vi "AdminLogInSearchHistory(SubVI).vi"() -> ()   [LabVIEW 2013]
uses:
  <vilib>/addons/database/Connection.llb/DB Tools Open Connec (String).vi
  <vilib>/addons/database/_DB Variant To Data/Database Variant To Data.xnode
  <vilib>/addons/database/NI_Database_API.lvlib
panel:
  in  "Search another student":bool
  in  "Confirm":bool
  in  "Student Admin No:":string
  in  "Go Back":bool
  out "Student Admin No: 2":string
  out "Array 2":string[][](array[string])
  out "AdminNo.Accepted?":string
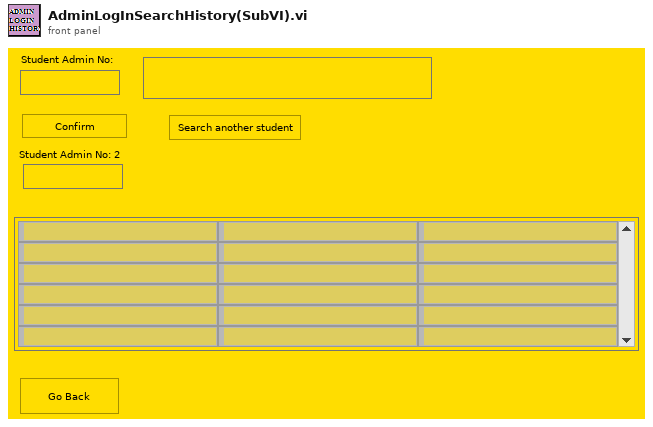
[diagram p1: front panel]
types:
  T1 = enum8{"Enabled", "Disabled", "Disabled and Grayed Out"}
  T2 = typedef "NI_Database_API.lvlib/Conn ObjectReference.ctl" = refnum<k1>
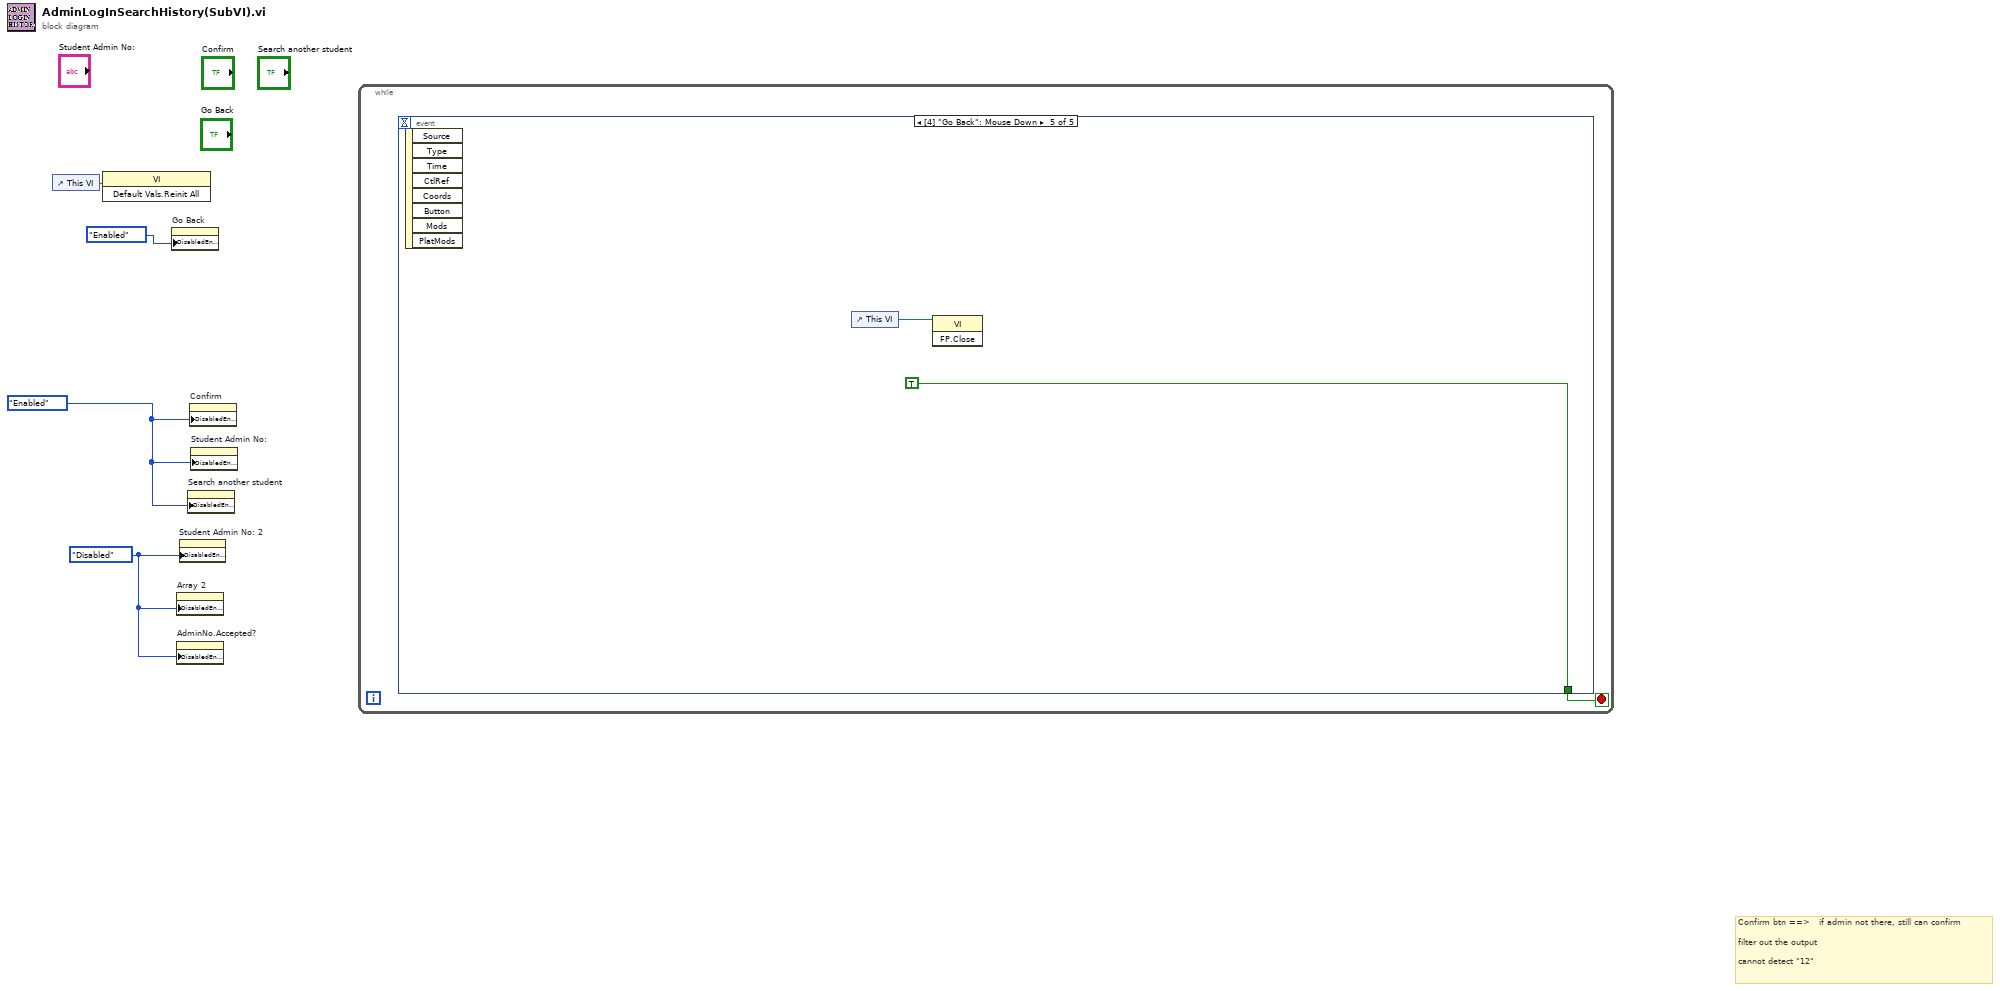
[diagram p0: block diagram]
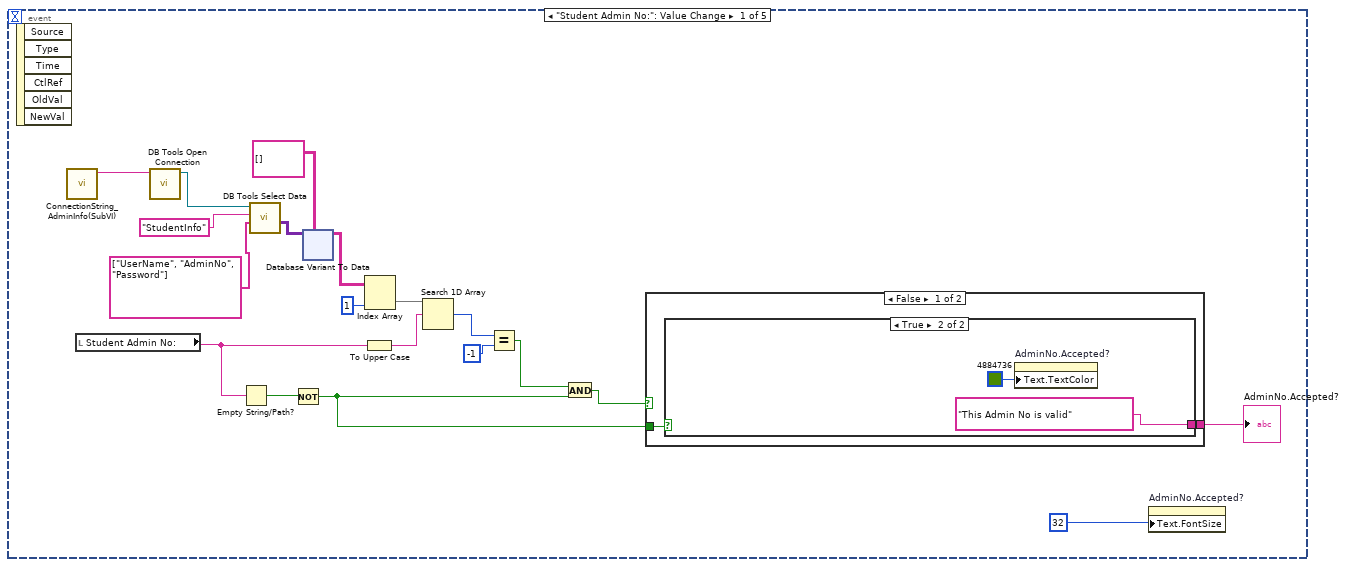
[diagram p2: hidden frame]
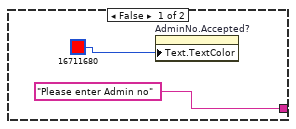
[diagram p3: hidden frame]
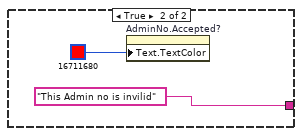
[diagram p4: hidden frame]
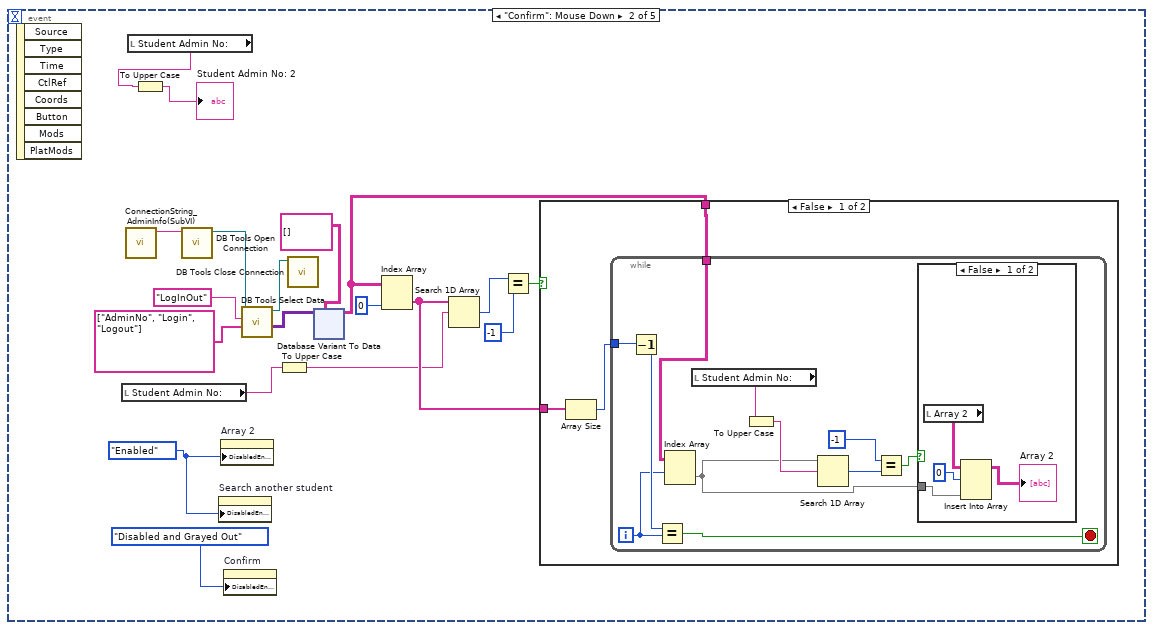
[diagram p5: hidden frame]
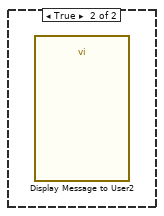
[diagram p7: hidden frame]
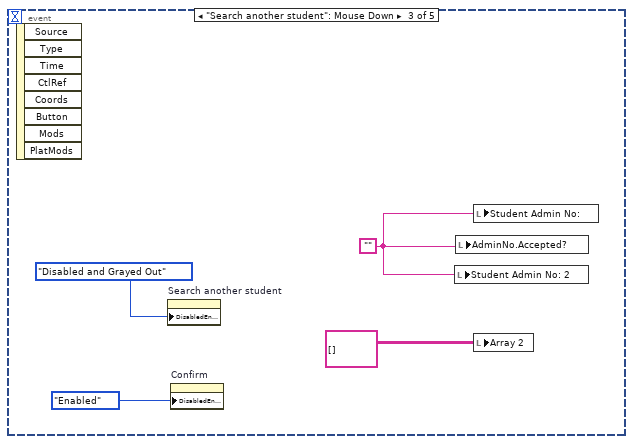
[diagram p8: hidden frame]
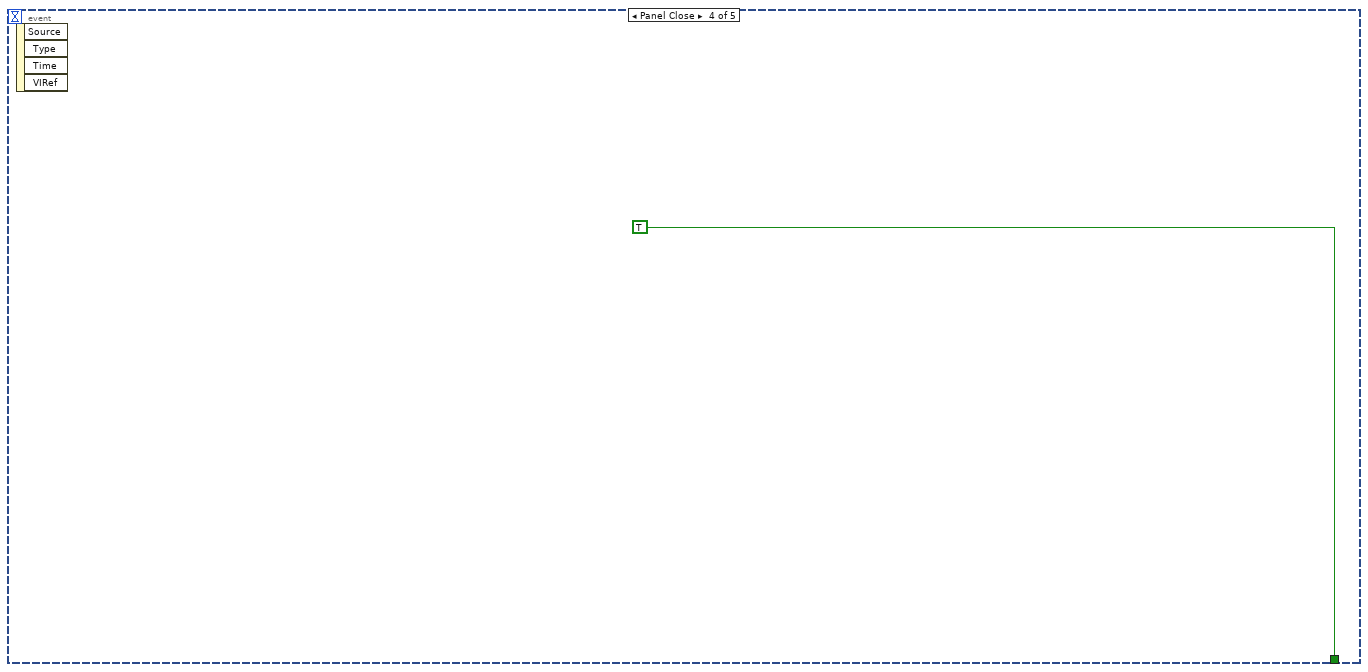
[diagram p9: hidden frame]
diagram:
  w3 = T1."Disabled"
  w1 = T1."Enabled"
  # "Confirm btn ==>   if admin not there, still can confirm\n\nfilter out the output\n\ncannot detect \"12\""
  n1 = control-ref of="This VI"() -> (w4:refnum<vi>)
  n2 = invoke class="VI" method="Default Vals.Reinit All"(reference=w4) -> ()  [unwired: 2 in, 3 out]
  n3 = property on="Go Back" class="Bool (strict)"("DisabledEnum"=T1."Enabled") -> ()  [unwired: 2 in, 2 out]
  n4 = property on="Array 2" class="Arr (strict)"("DisabledEnum"=w3) -> ()  [unwired: 2 in, 2 out]
  n5 = property on="AdminNo.Accepted?" class="Str"("DisabledEnum"=w3) -> ()  [unwired: 2 in, 2 out]
  n6 = property on="Student Admin No: 2" class="Str"("DisabledEnum"=w3) -> ()  [unwired: 2 in, 2 out]
  n7 = property on="Search another student" class="Bool (strict)"("DisabledEnum"=w1) -> ()  [unwired: 2 in, 2 out]
  n8 = property on="Confirm" class="Bool (strict)"("DisabledEnum"=w1) -> ()  [unwired: 2 in, 2 out]
  n9 = property on="Student Admin No:" class="Str"("DisabledEnum"=w1) -> ()  [unwired: 2 in, 2 out]
  n10 = while {
    stop <- w5 stop-if-true
    n11 = event shown="[4] \"Go Back\": Mouse Down" {
      selector: _ -> [_ _ _ _ _]
      dyn-events: _ -> [_ _ _ _ _]
      timeout: _ -> [_ _ _ _ _]
      tunnel: [_ _ _ TRUE TRUE] -> w5
      event "Student Admin No:": Value Change {
        n12 = event-data() -> ()  [unwired: 1 in, 6 out]
        n13 = call "ConnectionString_AdminInfo(SubVI).vi"() -> ("ConnectionString"=w22:string)  [unwired: 11 in]
        n14 = local read "Student Admin No:"() -> (w20:string)
        n15 = call-poly <vilib>:"DB Tools Open Connection.vi"("connection information"=w22) -> ("connection reference"=w23:T2)  [unwired: 7 in, 1 out]
        n16 = Empty String/Path?(string/path=w20) -> (empty?=w16:bool)
        n17 = call <vilib>:"DB Tools Select Data.vi"("columns"=string[] ["UserName", "AdminNo", "Password"], "table"="StudentInfo", "connection reference"=w23) -> ("data"=w9:variant[][])  [unwired: 3 in, 2 out]
        n18 = Not(x=w16) -> (.not. x?=w18:bool)
        n19 = xnode "Database Variant To Data"("database variant"=w9, "type"=string[][] []) -> ("data"=w10:string[][])  [unwired: 1 in, 1 out]
        n20 = To Upper Case(1:w20) -> (0:w13:string)
        n21 = Index Array(array=w10, index (col)=1) -> (element=w12:string[])  [unwired: 1 in]
        n22 = Search 1D Array(1D array=w12, element=w13) -> (index of element=w14:i32)  [unwired: 1 in]
        n23 = Equal?(x=w14, y=-1) -> (x = y?=w17:bool)
        n24 = And(x=w17, y=w18) -> (x .and. y?=w24:bool)
        n25 = case shown="False" w24 {
          tunnel: w18 -> [w25 _]
          tunnel: [w26 "This Admin no is invilid"] -> w19
          frame False {
            n26 = case shown="True" w25 {
              tunnel: ["Please enter Admin no" "This Admin No is valid"] -> w26
              frame False {
                n27 = property on="AdminNo.Accepted?" class="Str"("Text.TextColor"=u32 16711680) -> ()  [unwired: 2 in, 2 out]
              }
              frame True {
                n28 = property on="AdminNo.Accepted?" class="Str"("Text.TextColor"=u32 4884736) -> ()  [unwired: 2 in, 2 out]
              }
            }
          }
          frame True {
            n29 = property on="AdminNo.Accepted?" class="Str"("Text.TextColor"=u32 16711680) -> ()  [unwired: 2 in, 2 out]
          }
        }
        "AdminNo.Accepted?" <- w19
        n30 = property on="AdminNo.Accepted?" class="Str"("Text.FontSize"=32) -> ()  [unwired: 2 in, 2 out]
      }
      event "Confirm": Mouse Down {
        w94 = T1."Enabled"
        n31 = event-data() -> ()  [unwired: 1 in, 8 out]
        n32 = local read "Student Admin No:"() -> (w90:string)
        n33 = call "ConnectionString_AdminInfo(SubVI).vi"() -> ("ConnectionString"=w78:string)  [unwired: 11 in]
        n34 = local read "Student Admin No:"() -> (w86:string)
        n35 = To Upper Case(1:w86) -> (0:→"Student Admin No: 2":string)
        n36 = call-poly <vilib>:"DB Tools Open Connection.vi"("connection information"=w78) -> ("connection reference"=w77:T2)  [unwired: 7 in, 1 out]
        n37 = property on="Search another student" class="Bool (strict)"("DisabledEnum"=w94) -> ()  [unwired: 2 in, 2 out]
        n38 = property on="Array 2" class="Arr (strict)"("DisabledEnum"=w94) -> ()  [unwired: 2 in, 2 out]
        n39 = property on="Confirm" class="Bool (strict)"("DisabledEnum"=T1."Disabled and Grayed Out") -> ()  [unwired: 2 in, 2 out]
        n40 = call <vilib>:"DB Tools Select Data.vi"("columns"=string[] ["AdminNo", "Login", "Logout"], "table"="LogInOut", "connection reference"=w77) -> ("data"=w83:variant[][], "connection reference out"=w81:T2)  [unwired: 3 in, 1 out]
        n41 = To Upper Case(1:w90) -> (0:w85:string)
        n42 = call <vilib>:"DB Tools Close Connection.vi"("connection reference"=w81) -> ()  [unwired: 6 in, 1 out]
        n43 = xnode "Database Variant To Data"("database variant"=w83, "type"=string[][] []) -> ("data"=w92:string[][])  [unwired: 1 in, 1 out]
        n44 = Index Array(array=w92, index (col)=0 ("disabled index (col)")) -> (element=w93:string[])  [unwired: 1 in]
        n45 = Search 1D Array(1D array=w93, element=w85) -> (index of element=w91:i32)  [unwired: 1 in]
        n46 = Equal?(x=w91, y=-1) -> (x = y?=w80:bool)
        n47 = case shown="False" w80 {
          tunnel: w92 -> [w142 _]
          tunnel: w93 -> [w140 _]
          frame False {
            n48 = Array Size(array=w140) -> (size(s)=w141:i32)
            n49 = while {
              tunnel: w141 -> [w152]
              tunnel: w142 -> [w149]
              i -> [w150]
              stop <- w153 stop-if-true
              n50 = Decrement(x=w152) -> (x-1=w151:i32)
              n51 = Equal?(x=w151, y=w150) -> (x = y?=w153:bool)
              n52 = Index Array(array=w149, index (row)=w150) -> (element=w145:string[])  [unwired: 1 in]
              n53 = local read "Student Admin No:"() -> (w148:string)
              n54 = To Upper Case(1:w148) -> (0:w147:string)
              n55 = Search 1D Array(1D array=w145, element=w147) -> (index of element=w144:i32)  [unwired: 1 in]
              n56 = Equal?(x=-1, y=w144) -> (x = y?=w146:bool)
              n57 = case shown="False" w146 {
                tunnel: w145 -> [w154 _]
                frame False {
                  n58 = local read "Array 2"() -> (w156:string[][])
                  n59 = Insert Into Array(array=w156, index (row)=0, new element=w154) -> (→"Array 2":string[][])  [unwired: 1 in]
                }
                frame True {
                }
              }
            }
          }
          frame True {
            n60 = call "Display Message to User2"() -> ()  [unwired: 10 in, 2 out]
          }
        }
      }
      event "Search another student": Mouse Down {
        w159 = ""
        n61 = event-data() -> ()  [unwired: 1 in, 8 out]
        n62 = property on="Search another student" class="Bool (strict)"("DisabledEnum"=T1."Disabled and Grayed Out") -> ()  [unwired: 2 in, 2 out]
        n63 = property on="Confirm" class="Bool (strict)"("DisabledEnum"=T1."Enabled") -> ()  [unwired: 2 in, 2 out]
        n64 = local write "Student Admin No: 2"(w159) -> ()
        n65 = local write "AdminNo.Accepted?"(w159) -> ()
        n66 = local write "Student Admin No:"(w159) -> ()
        n67 = local write "Array 2"(string[][] []) -> ()
      }
      event Panel Close {
        n68 = event-data() -> ()  [unwired: 1 in, 4 out]
      }
      event "Go Back": Mouse Down {
        n69 = event-data() -> ()  [unwired: 1 in, 8 out]
        n70 = control-ref of="This VI"() -> (w164:refnum<vi>)
        n71 = invoke class="VI" method="FP.Close"(reference=w164) -> ()  [unwired: 2 in, 3 out]
      }
    }
  }
